vi "Count Num of True Element in 3D Array.vi"(8 "错误输入":errorcluster, 10 "Mode":enum16{"Row", "Col"}(ring), 11 "3D Boolean Array":bool[][][](array[boolean])) -> (0 "错误输出":errorcluster, 3 "Num of True":i16[][](array[numeric]))   [LabVIEW 2011]
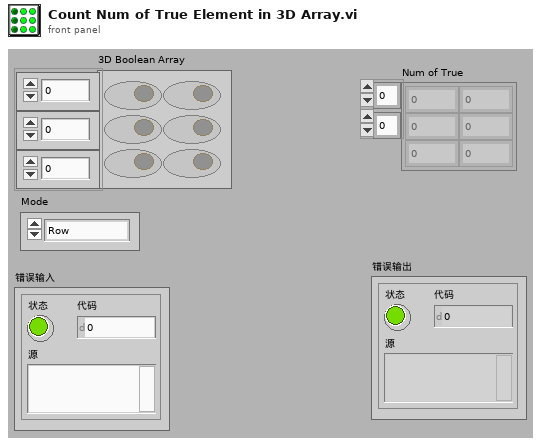
[diagram p1: front panel]
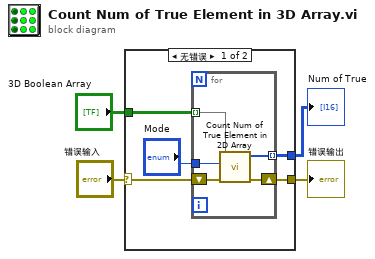
[diagram p0: block diagram]
diagram:
  n1 = case shown="无错误" "错误输入" {
    selector: "错误输入" -> [w9 w15]
    tunnel: [w7 w15] -> w3
    tunnel: "3D Boolean Array" -> [w6 _]
    tunnel: [w8 _] -> w1
    frame No Error {
      n2 = for {
        shift-right: [w13] -> w7
        shift-left: w9 -> [w14]
        tunnel: [w12] -> w8 mode=indexing
        tunnel: w6 -> [w11] mode=indexing
        tunnel: "Mode" -> [w10]
        n3 = call "Count Num of True Element in 2D Array.vi"("错误输入"=w14, "Mode"=w10, "2D Boolean Array"=w11) -> ("错误输出"=w13:errorcluster, "Num of True"=w12:i16[])  [unwired: 7 in]
      }
    }
    frame Error {
    }
  }
  "错误输出" <- w3
  "Num of True" <- w1
